vi "FoodLogic.vi"(11 "Level input":u32[][](array[colorbox])) -> (1 "X Position":i32, 2 "Y Position":i32, 3 "Level output":u32[][](array[colorbox]), 4 "Pixel Occupied?":bool)   [LabVIEW 2021]
uses:
  GlobalVariables/Board_Colors.vi
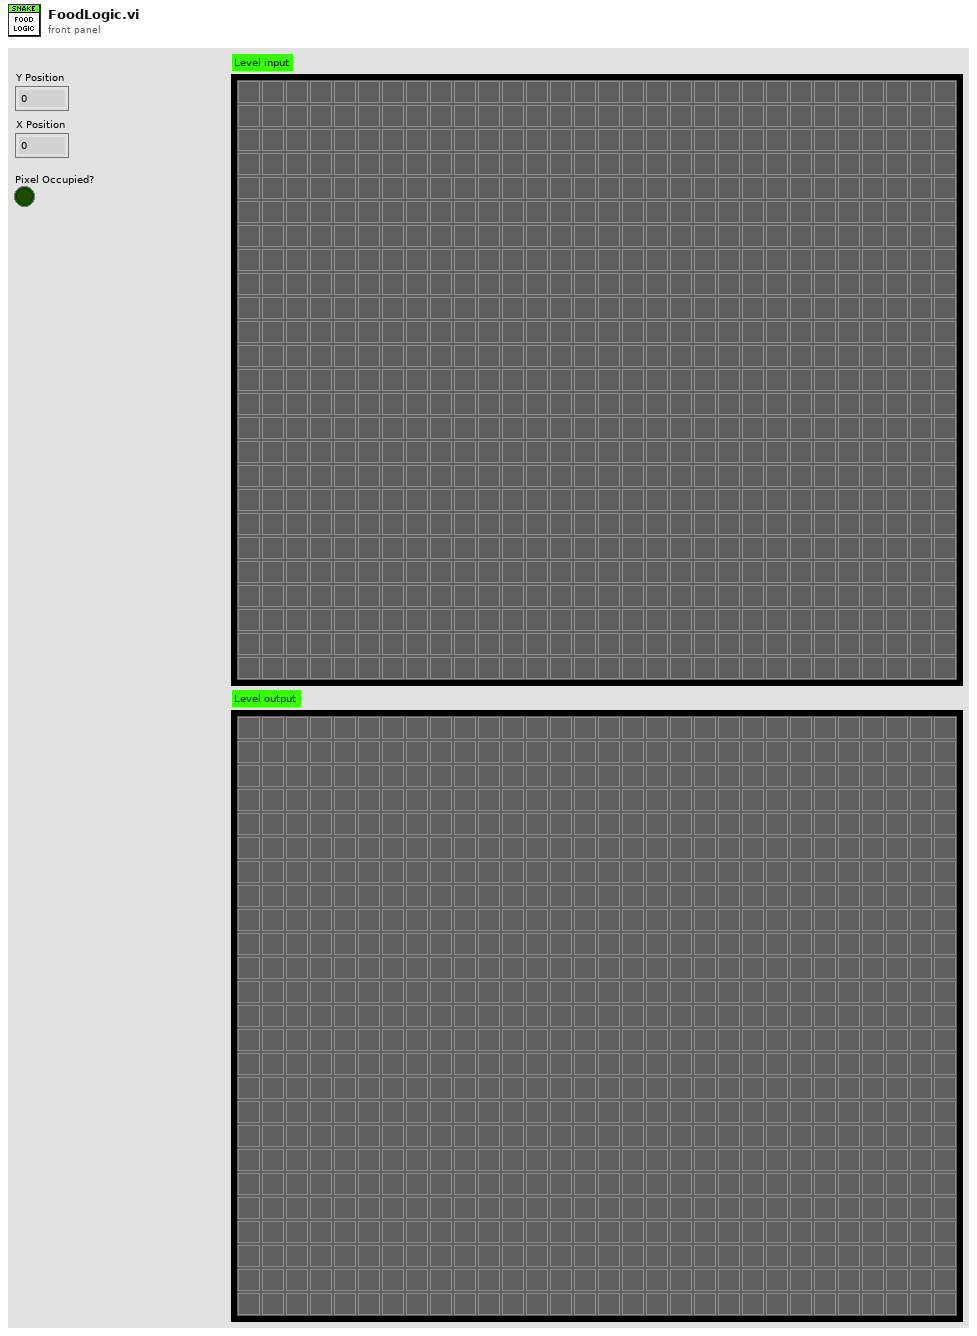
[diagram p1: front panel]
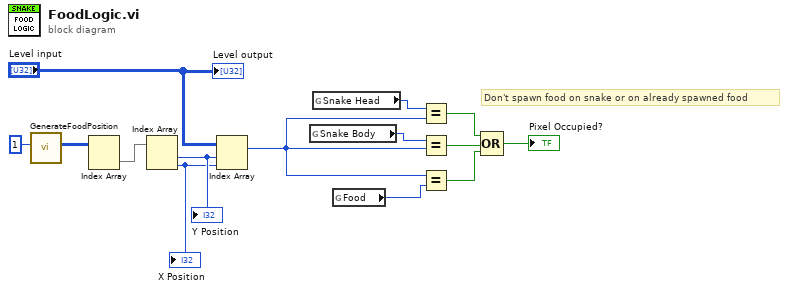
[diagram p0: block diagram]
diagram:
  # "Don't spawn food on snake or on already spawned food"
  n1 = call "GenerateFoodPosition.vi"("Food Amount"=1) -> ("Food Array"=w13:i32[][])  [unwired: 10 in]
  n2 = Index Array(array=w13) -> (element=w12:i32[])  [unwired: 2 in]
  n3 = Index Array(array=w12) -> (element #1=w11:i32, element #2=w9:i32)  [unwired: 2 in]
  "X Position" <- w9
  "Y Position" <- w11
  n4 = Index Array(array="Level input", index (row)=w11, index (col)=w9) -> (element=w4:u32)
  n5 = global read "Board_Colors.vi" "Snake Body"() -> (w1:u32)
  n6 = global read "Board_Colors.vi" "Snake Head"() -> (w2:u32)
  n7 = global read "Board_Colors.vi" "Food"() -> (w3:u32)
  n8 = Equal?(x=w2, y=w4) -> (x = y?=w7:bool)
  n9 = Equal?(x=w1, y=w4) -> (x = y?=w8:bool)
  n10 = Equal?(x=w4, y=w3) -> (x = y?=w6:bool)
  n11 = Compound Arithmetic op=OR(w7, w8, w6) -> (→"Pixel Occupied?":bool)
  "Level output" <- "Level input"
